vi "Get Trajectory Mode.vi"(4 "error in (no error)":errorcluster, 6 "Axis (1)":i32=1 min=1 max=3, 7 "VISA resource name":refnum<visa-resource-name>) -> (0 "error out":errorcluster, 2 "Trajectory Mode":T1(ring), 3 "VISA resource name out":refnum<visa-resource-name>)   [LabVIEW 2015, in "Newport ESP301.lvlib"]
doc: "This command gets the trajectory mode <B>Tajectory Mode</B> on the axis specified by <B>Axis (1)</B>."
uses:
  Newport ESP301.lvlib
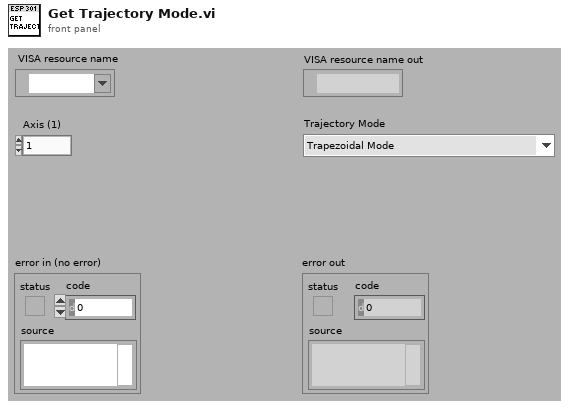
[diagram p1: front panel]
types:
  T1 = enum16{"Trapezoidal Mode", "S-curve Mode", "Jog Mode", "Slave to master's desired position (trajectory)", "Slave to master's actual position (feedback)", "Slave to master's actual velocity for jogging"}
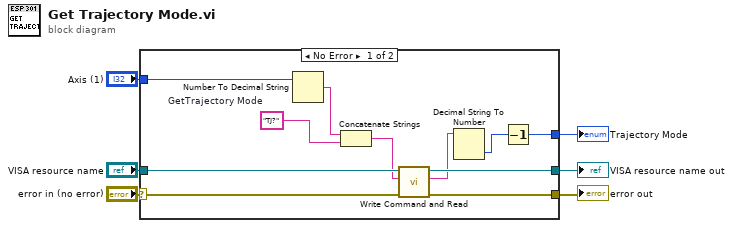
[diagram p0: block diagram]
diagram:
  n1 = case shown="No Error" "error in (no error)" {
    selector: "error in (no error)" -> [w16 w19]
    tunnel: [w15 w19] -> w5
    tunnel: "VISA resource name" -> [w17 w18]
    tunnel: [w14 w18] -> w3
    tunnel: "Axis (1)" -> [w11 _]
    tunnel: [w7 _] -> w1
    frame No Error {
      w13 = "TJ?"  # GetTrajectory Mode
      n2 = Number To Decimal String(number=w11) -> (decimal integer string=w12:string)  [unwired: 1 in]
      n3 = Concatenate Strings(w12, w13) -> (w10:string)
      n4 = call "Write Command and Read.vi"("error in (no error)"=w16, "Command"=w10, "VISA resource name"=w17) -> ("error out"=w15:errorcluster, "Returned string"=w9:string, "VISA resource name out"=w14:refnum<visa-resource-name>)  [unwired: 4 in]
      n5 = Decimal String To Number(string=w9) -> (number=w8:i32)  [unwired: 2 in, 1 out]
      n6 = Decrement(x=w8) -> (x-1=w7:i32)
    }
    frame Error {
    }
  }
  "error out" <- w5
  "VISA resource name out" <- w3
  "Trajectory Mode" <- w1
